vi "ZC_jiben.vi"(0 "action":string, 1 "LabVIEW Web Service Request":refnum<class "Web Request.lvclass"> caption="LabVIEW Web服务请求", 3 "pinpai":string, 4 "xinghao":string, 5 "id":string, 6 "beizhu":string, 8 "key":string, 9 "name":string, 11 "yjleibie":string, 12 "ejleibie":string, 14 "shchsh":string, 15 "number":string) -> (10 "error":errorcluster)   [LabVIEW 2017]
uses:
  <vilib>/wsapi/Web Request.lvclass
panel:
  out "postdata":string caption="post数据"
  out "error out":errorcluster caption="错误输出"
  # "Web服务请求输入接线端用于调用“Web服务”选板的VI。除非不需要访问该选板，否则不要在连线板上删除这个输入接线端。"
  # "添加至连线板的每一个其他输入控件，在URL中对应于一个输入。如需在接线端模式输出（默认设置）下包含显示控件，则该显示控件必须与连线板相连。"
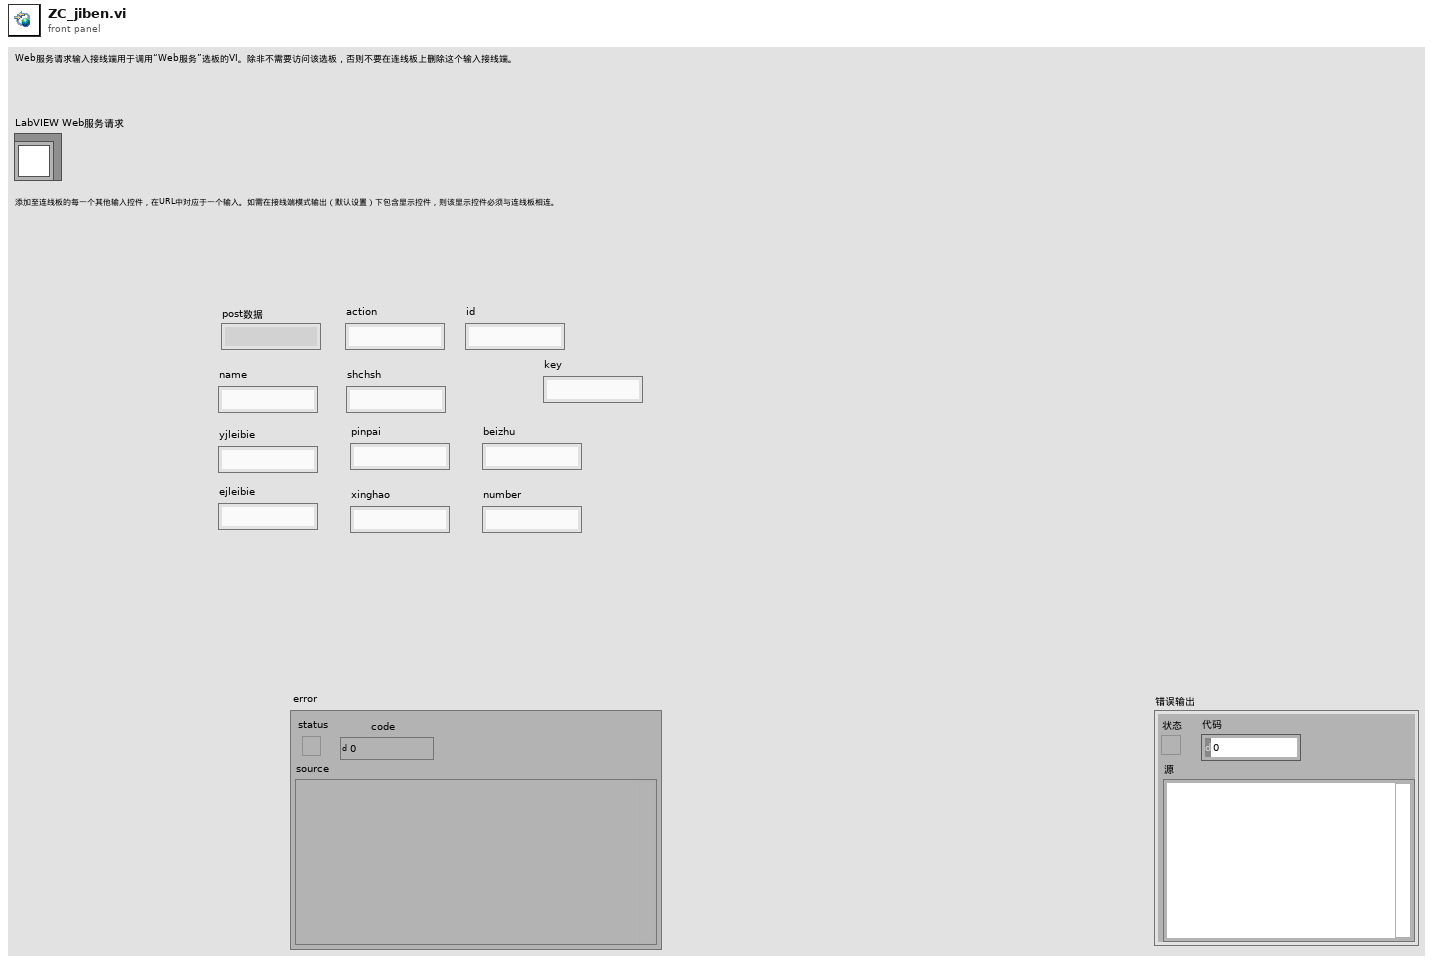
[diagram p1: front panel]
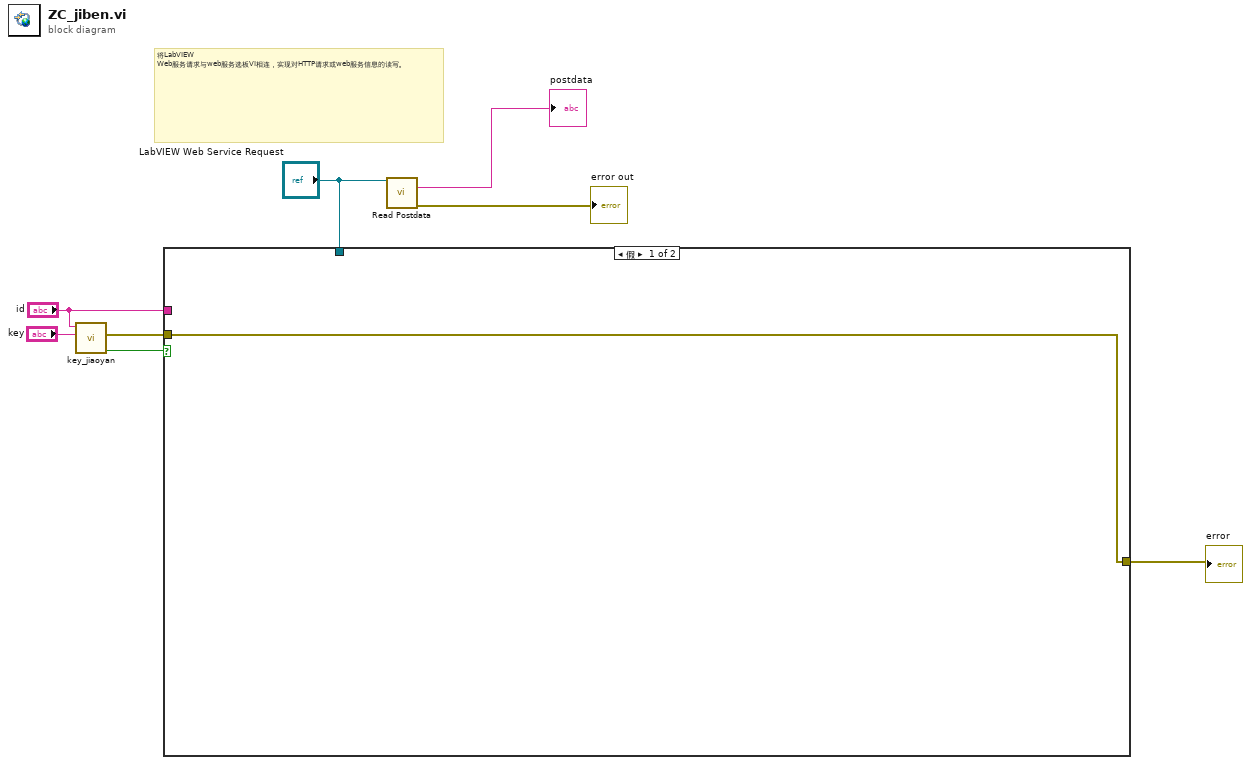
[diagram p0: block diagram]
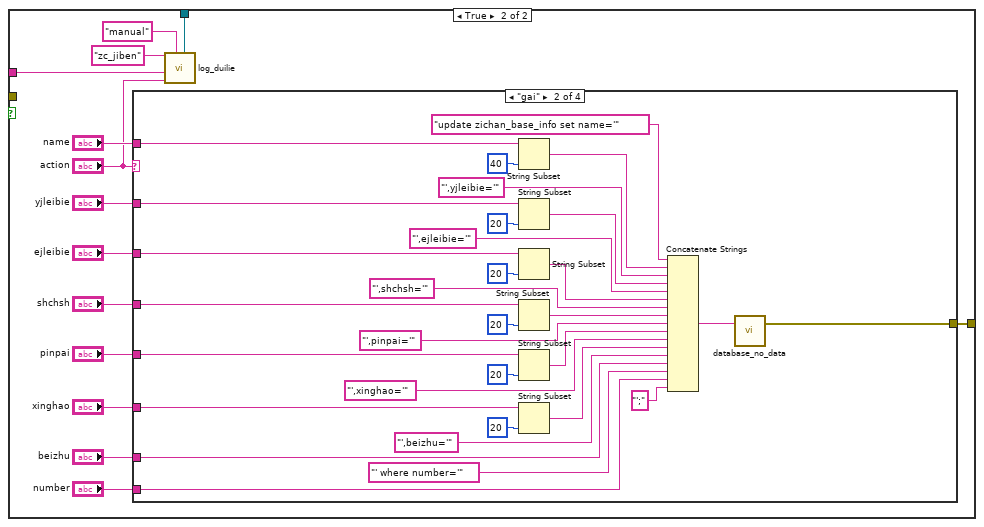
[diagram p2: hidden frame]
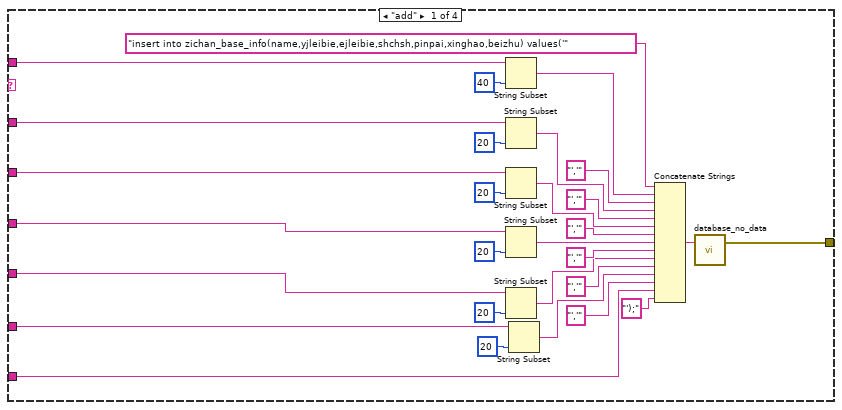
[diagram p3: hidden frame]
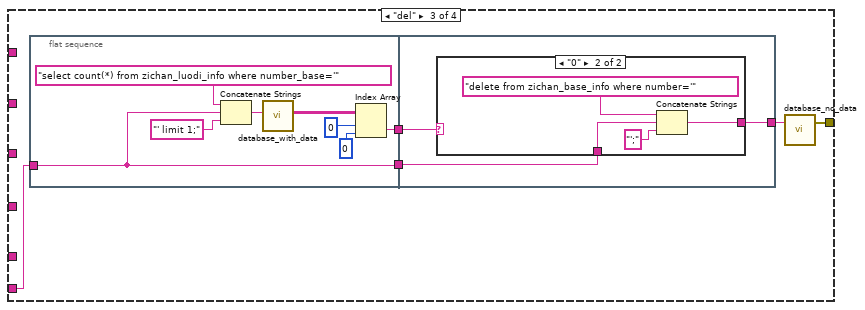
[diagram p4: hidden frame]
diagram:
  # "将LabVIEW Web服务请求与web服务选板VI相连，实现对HTTP请求或web服务信息的读写。"
  n1 = call "key_jiaoyan.vi"("key_client"="key", "gonghao"="id") -> ("jy"=w2:bool, "error"=w1:errorcluster)  [unwired: 8 in]
  n2 = case shown="假" w2 {
    tunnel: [w9 w23] -> w7
    tunnel: "LabVIEW Web Service Request" -> [_ w12]
    tunnel: "id" -> [_ w10]
    tunnel: w1 -> [w9 _]
    frame False {
    }
    frame True {
      n3 = case shown="\"gai\"" "action" {
        tunnel: [w31 w63 w88 _] -> w23
        tunnel: "name" -> [w30 w62 _ _]
        tunnel: "yjleibie" -> [w29 w61 _ _]
        tunnel: "ejleibie" -> [w28 w60 _ _]
        tunnel: "shchsh" -> [w27 w59 _ _]
        tunnel: "pinpai" -> [w26 w58 _ _]
        tunnel: "xinghao" -> [w25 w57 _ _]
        tunnel: "beizhu" -> [w24 w56 _ _]
        tunnel: "number" -> [_ w54 w85 _]
        frame "add" {
          n4 = String Subset(string=w30, length (rest)=40 ("长度（剩余）")) -> (substring=w48:string)  [unwired: 1 in]
          n5 = String Subset(string=w29, length (rest)=20 ("长度（剩余）")) -> (substring=w46:string)  [unwired: 1 in]
          n6 = String Subset(string=w28, length (rest)=20 ("长度（剩余）")) -> (substring=w44:string)  [unwired: 1 in]
          n7 = String Subset(string=w27, length (rest)=20 ("长度（剩余）")) -> (substring=w42:string)  [unwired: 1 in]
          n8 = String Subset(string=w26, length (rest)=20 ("长度（剩余）")) -> (substring=w37:string)  [unwired: 1 in]
          n9 = String Subset(string=w25, length (rest)=20 ("长度（剩余）")) -> (substring=w34:string)  [unwired: 1 in]
          n10 = Concatenate Strings("insert into zichan_base_info(name,yjleibie,ejleibie,shchsh,pinpai,xinghao,beizhu) values('" ("格式字符串"), w48, "','" ("字符串"), w46, "','" ("字符串"), w44, "','" ("字符串"), w42, "','" ("字符串"), w37, "','" ("字符串"), w34, "','" ("字符串"), w24, "');" ("字符串")) -> (w32:string)
          n11 = call "database_no_data.vi"("input"=w32) -> ("error"=w31:errorcluster)  [unwired: 2 in]
        }
        frame "gai" {
          n12 = String Subset(string=w62, length (rest)=40 ("长度（剩余）")) -> (substring=w79:string)  [unwired: 1 in]
          n13 = String Subset(string=w61, length (rest)=20 ("长度（剩余）")) -> (substring=w77:string)  [unwired: 1 in]
          n14 = String Subset(string=w60, length (rest)=20 ("长度（剩余）")) -> (substring=w75:string)  [unwired: 1 in]
          n15 = String Subset(string=w59, length (rest)=20 ("长度（剩余）")) -> (substring=w73:string)  [unwired: 1 in]
          n16 = String Subset(string=w58, length (rest)=20 ("长度（剩余）")) -> (substring=w68:string)  [unwired: 1 in]
          n17 = String Subset(string=w57, length (rest)=20 ("长度（剩余）")) -> (substring=w66:string)  [unwired: 1 in]
          n18 = Concatenate Strings("update zichan_base_info set name='" ("格式字符串"), w79, "',yjleibie='" ("字符串"), w77, "',ejleibie='" ("字符串"), w75, "',shchsh='" ("字符串"), w73, "',pinpai='" ("字符串"), w68, "',xinghao='" ("字符串"), w66, "',beizhu='" ("字符串"), w56, "' where number='" ("字符串"), w54, "';" ("字符串")) -> (w64:string)
          n19 = call "database_no_data.vi"("input"=w64) -> ("error"=w63:errorcluster)  [unwired: 2 in]
        }
        frame "del" {
          n20 = flat-sequence {
            tunnel: w85 -> [w94]
            tunnel: [w94] -> w87
            tunnel: [w89] -> w86
            tunnel: [w99] -> w84
            tunnel: w87 -> [w98]
            tunnel: w86 -> [w97]
            frame #0 {
              n21 = Concatenate Strings("select count(*) from zichan_luodi_info where number_base='" ("格式字符串"), w94, "' limit 1;" ("字符串")) -> (w93:string)
              n22 = call "database_with_data.vi"("input"=w93) -> ("Data"=w90:string[][])  [unwired: 9 in, 1 out]
              n23 = Index Array(array=w90, index (row)=0 ("索引 (行)"), index (col)=0 ("禁用的索引 (列)")) -> (element=w89:string)
            }
            frame #1 {
              n24 = case shown="\"0\"" w97 {
                tunnel: [_ w101] -> w99
                tunnel: w98 -> [_ w100]
                frame "假", Default {
                }
                frame "0" {
                  n25 = Concatenate Strings("delete from zichan_base_info where number='" ("格式字符串"), w100, "';" ("字符串")) -> (w101:string)
                }
              }
            }
          }
          n26 = call "database_no_data.vi"("input"=w84) -> ("error"=w88:errorcluster)  [unwired: 2 in]
        }
        frame Default {
        }
      }
      n27 = call "log_duilie.vi"("LabVIEW Web Service Request"=w12, "type"="manual", "action"="action", "user"=w10, "yw"="zc_jiben") -> ()  [unwired: 7 in]
    }
  }
  "error" <- w7
  n28 = call <vilib>:"Read Postdata.vi"("LabVIEW Web Service Request"="LabVIEW Web Service Request") -> ("postdata"=→"postdata":string, "error out"=→"error out":errorcluster)  [unwired: 12 in, 1 out]
